vi "DisplayTableFilter.vi"(8 "Error In":errorcluster, 11 "DataPack Array":T1(array[cluster])) -> (0 "Error out":errorcluster, 2 "Propertynames":string[](array[string]), 3 "Table Array":string[][](array[string]))   [LabVIEW 2014]
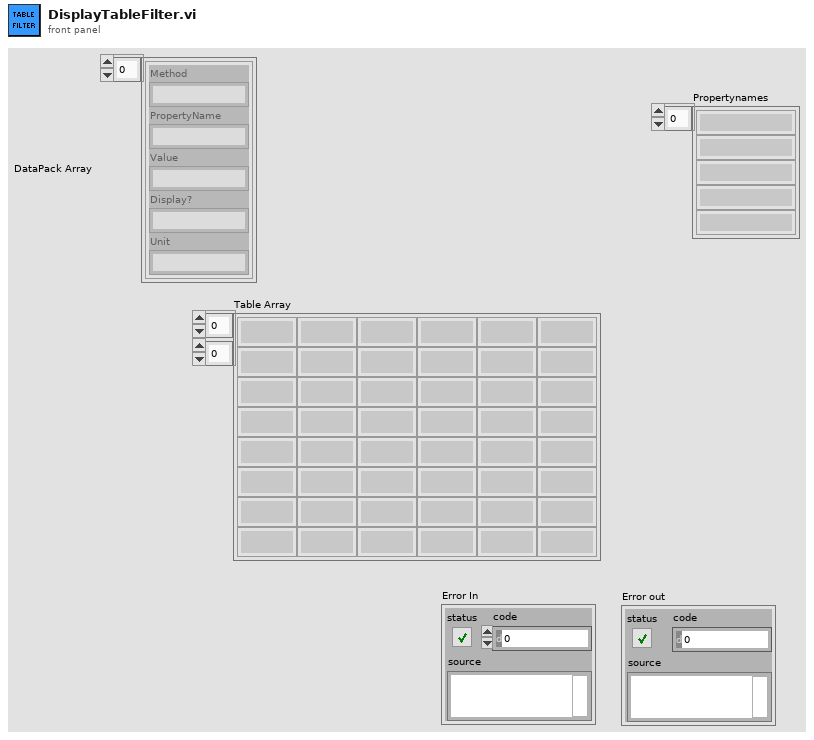
[diagram p1: front panel]
types:
  T1 = cluster{"Method":string, "PropertyName":string, "Value":string, "Display?":string, "Unit":string}[]
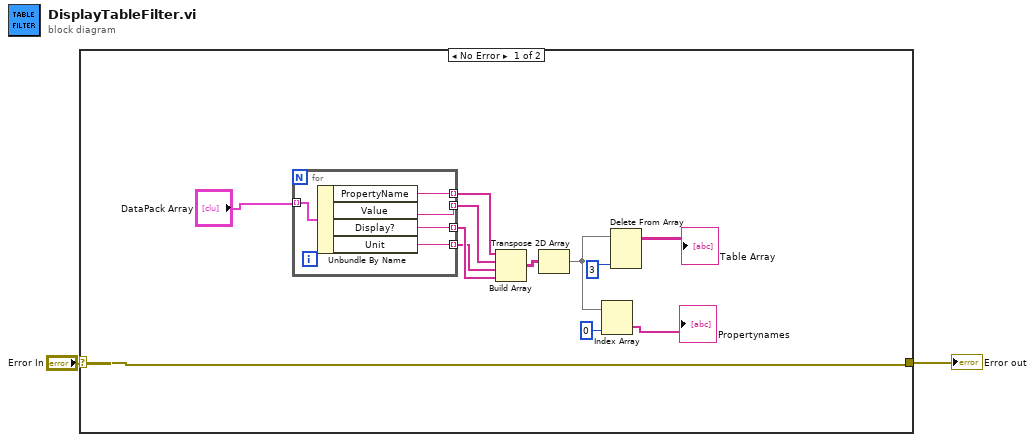
[diagram p0: block diagram]
diagram:
  n1 = case shown="No Error" "Error In" {
    selector: "Error In" -> [w10 w20]
    tunnel: [w10 w20] -> w2
    frame No Error {
      n2 = for {
        tunnel: "DataPack Array" -> [w19] mode=indexing
        tunnel: [w18] -> w14 mode=indexing
        tunnel: [w17] -> w12 mode=indexing
        tunnel: [w16] -> w4 mode=indexing
        tunnel: [w15] -> w3 mode=indexing
        n3 = Unbundle By Name(w19) -> ("PropertyName"=w17:string, "Value"=w18:string, "Display?"=w16:string, "Unit"=w15:string)
      }
      n4 = Build Array(w12, w14, w3, w4) -> (w13:string[][])
      n5 = Transpose 2D Array(2D array=w13) -> (transposed array=w7:string[][])
      n6 = Index Array(array=w7, index (col)=0 ("disabled index (col)")) -> (element=→"Propertynames":string[])  [unwired: 1 in]
      n7 = Delete From Array(array=w7, index (col)=3 ("disabled index (col)")) -> (array with subset deleted=→"Table Array":string[][])  [unwired: 2 in, 1 out]
    }
    frame Error {
    }
  }
  "Error out" <- w2
